vi "createObserverEvent.vi"(8 "error in":errorcluster, 9 "ObservableValue":variant[](array[variant]), 10 "ObservableName":string[](array[string]), 11 "ObserverClass in":refnum<class "ObserverClass.lvclass">) -> (0 "error out":errorcluster, 3 "ObserverClass out":refnum<class "ObserverClass.lvclass">, 4 "size":i32)   [LabVIEW 2025, in "ObserverClass.lvlib" / "ObserverClass.lvclass"]
doc: "Create Observer Event for the input ObservableData"
uses:
  ObserverClass.lvclass
  ObserverClass.lvclass/ObserverClass.ctl
  ObserverClass.lvlib
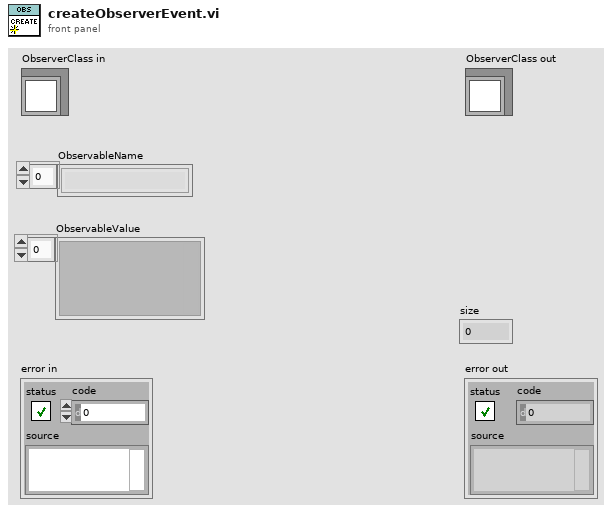
[diagram p1: front panel]
types:
  T1 = enum16{"Get", "Set", "Init", "Remove", "Destroy"}
  T2 = map{string, cluster{"ObserverEvent":refnum<user-event>, "ObserverNr":u64, "Value":variant}}
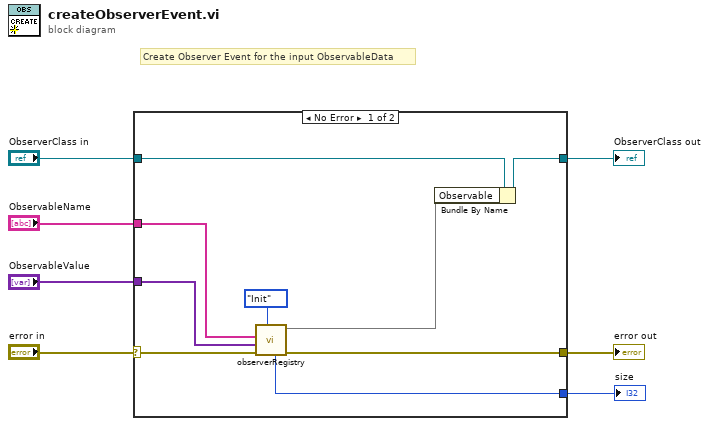
[diagram p0: block diagram]
diagram:
  # "Create Observer Event for the input ObservableData"
  n1 = case shown="No Error" "error in" {
    selector: "error in" -> [w12 w18]
    tunnel: [w14 w18] -> w6
    tunnel: [w16 w17] -> w4
    tunnel: "ObserverClass in" -> [w13 w17]
    tunnel: [w8 _] -> w3
    tunnel: "ObservableName" -> [w11 _]
    tunnel: "ObservableValue" -> [w10 _]
    frame No Error {
      n2 = call "observerRegistry.vi"("Action"=T1."Init", "error in"=w12, "ObservableValue"=w10, "ObservableName"=w11) -> ("error out"=w14:errorcluster, "Observable out"=w9:T2, "size"=w8:i32)  [unwired: 5 in]
      n3 = Bundle By Name(cluster=w13, "Observable"=w9) -> (w16:refnum<class "ObserverClass.lvclass">)
    }
    frame Error {
    }
  }
  "error out" <- w6
  "ObserverClass out" <- w4
  "size" <- w3
